vi "Serialize Properties.vi"(8 "error in (no error)":errorcluster, 10 "Properties":refnum<class "Property.lvclass">[](array[class]), 11 "Node in":refnum<k20>) -> (0 "error out":errorcluster, 3 "Node out":refnum<k20>)   [LabVIEW 2013, in "JUnit XML.lvlib" / "Test Suite.lvclass"]
uses:
  Test Suite.lvclass
  Property/Property.lvclass
  <vilib>/xml/Close Reference(Node).vi
  <vilib>/xml/NI_XML.lvlib
  XML/XML.lvlib
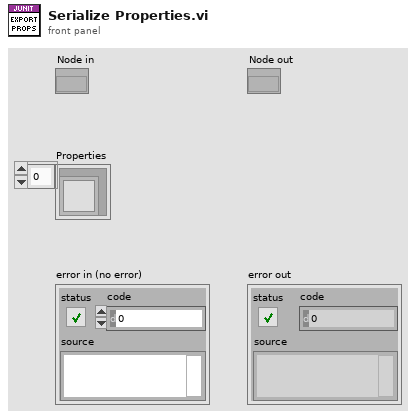
[diagram p1: front panel]
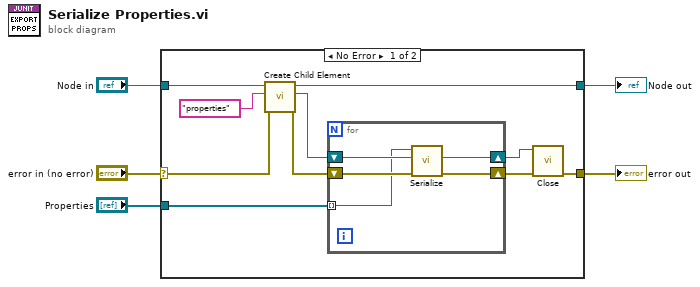
[diagram p0: block diagram]
diagram:
  n1 = case shown="No Error" "error in (no error)" {
    selector: "error in (no error)" -> [w6 w22]
    tunnel: "Node in" -> [w15 w21]
    tunnel: [w13 w22] -> w4
    tunnel: [w12 w21] -> w3
    tunnel: "Properties" -> [w9 _]
    frame No Error {
      n2 = call "Create Child Element.vi"("error in (no error)"=w6, "Name"="properties" ("Tag Name"), "Element in"=w15) -> ("error out"=w11:errorcluster, "Child Element"=w10:refnum<k20>, "Element out"=w12:refnum<k20>)  [unwired: 6 in]
      n3 = for {
        shift-right: [w19] -> w8
        shift-left: w10 -> [w20]
        shift-right: [w18] -> w7
        shift-left: w11 -> [w17]
        tunnel: w9 -> [w16] mode=indexing
        n4 = call "Serialize.vi"("error in (no error)"=w17, "Element in"=w20, "Property in"=w16) -> ("error out"=w18:errorcluster, "Element out"=w19:refnum<k20>)  [unwired: 6 in, 1 out]
      }
      n5 = call-poly <vilib>:"Close.vi"("error in (no error)"=w7, "node"=w8) -> ("error out"=w13:errorcluster)  [unwired: 7 in]
    }
    frame Error {
    }
  }
  "error out" <- w4
  "Node out" <- w3
